vi "SR 8XX read Channel 1&2_Scale.vi"(5 "enable auto?":bool, 6 "read data":enum16{"None", "X Y", "X only"}(ring), 7 "830":bool, 8 "channel":enum16{"R ", "X channel only", "Y channel only"}(ring), 9 "parameters_x":dbl[](array[numeric])=[1.0, 0.95, 0.05, 1e-07, 0.0] format="%.2e", 10 "Point #":i32, 11 "Instrument Address":refnum<visa-resource-name>="GPIB1::4::INSTR") -> (0 "changed range":u8, 1 "changed":bool, 2 "Data":dbl[](array[numeric]) format="%.2e", 3 "CH Output":dbl[](array[numeric]) format="%.2e", 4 "error in (no error) 2":errorcluster)   [LabVIEW 2019]
doc: "This VI reads two channels of the PAR 5210 lockin. It will not work for the 5208. The output is an array of values. The input is the numeric GPIB address.\nScott Hannahs, F. Bitter National Magnet Lab, May 1993"
panel:
  out "original sensitivity":dbl format="%#_2e"
  out "In range":bool
  out "lower limit":dbl format="%#_6e"
  out "upper limit":dbl format="%#_6e"
  out "Y-chanel AO":dbl format="%#_3e"
  out "X-chanel AO":dbl format="%#_3e"
  out "signal > sensitivity":bool
  # "865"
  # "lowest\nsensitivity"
  # "upper\nlimit"
  # "lower\nlimit"
  # "wait after change(sec)"
  # "out of range"
  # "signal < sensitivity"
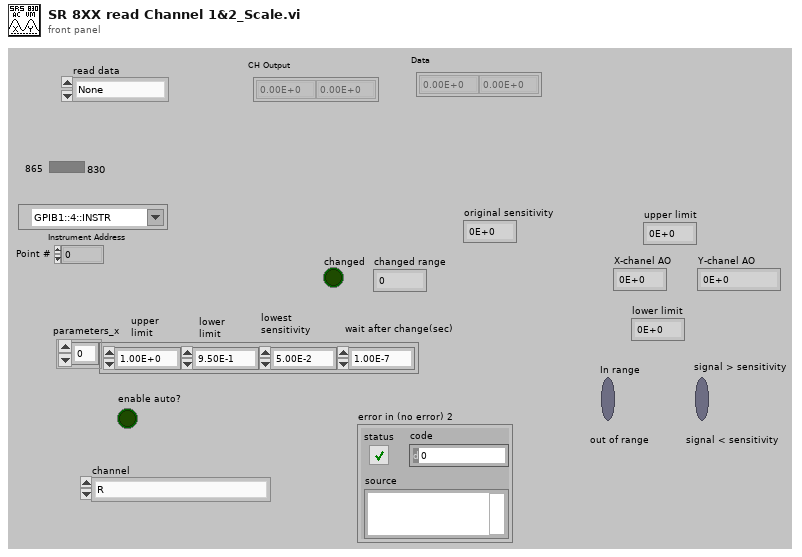
[diagram p1: front panel]
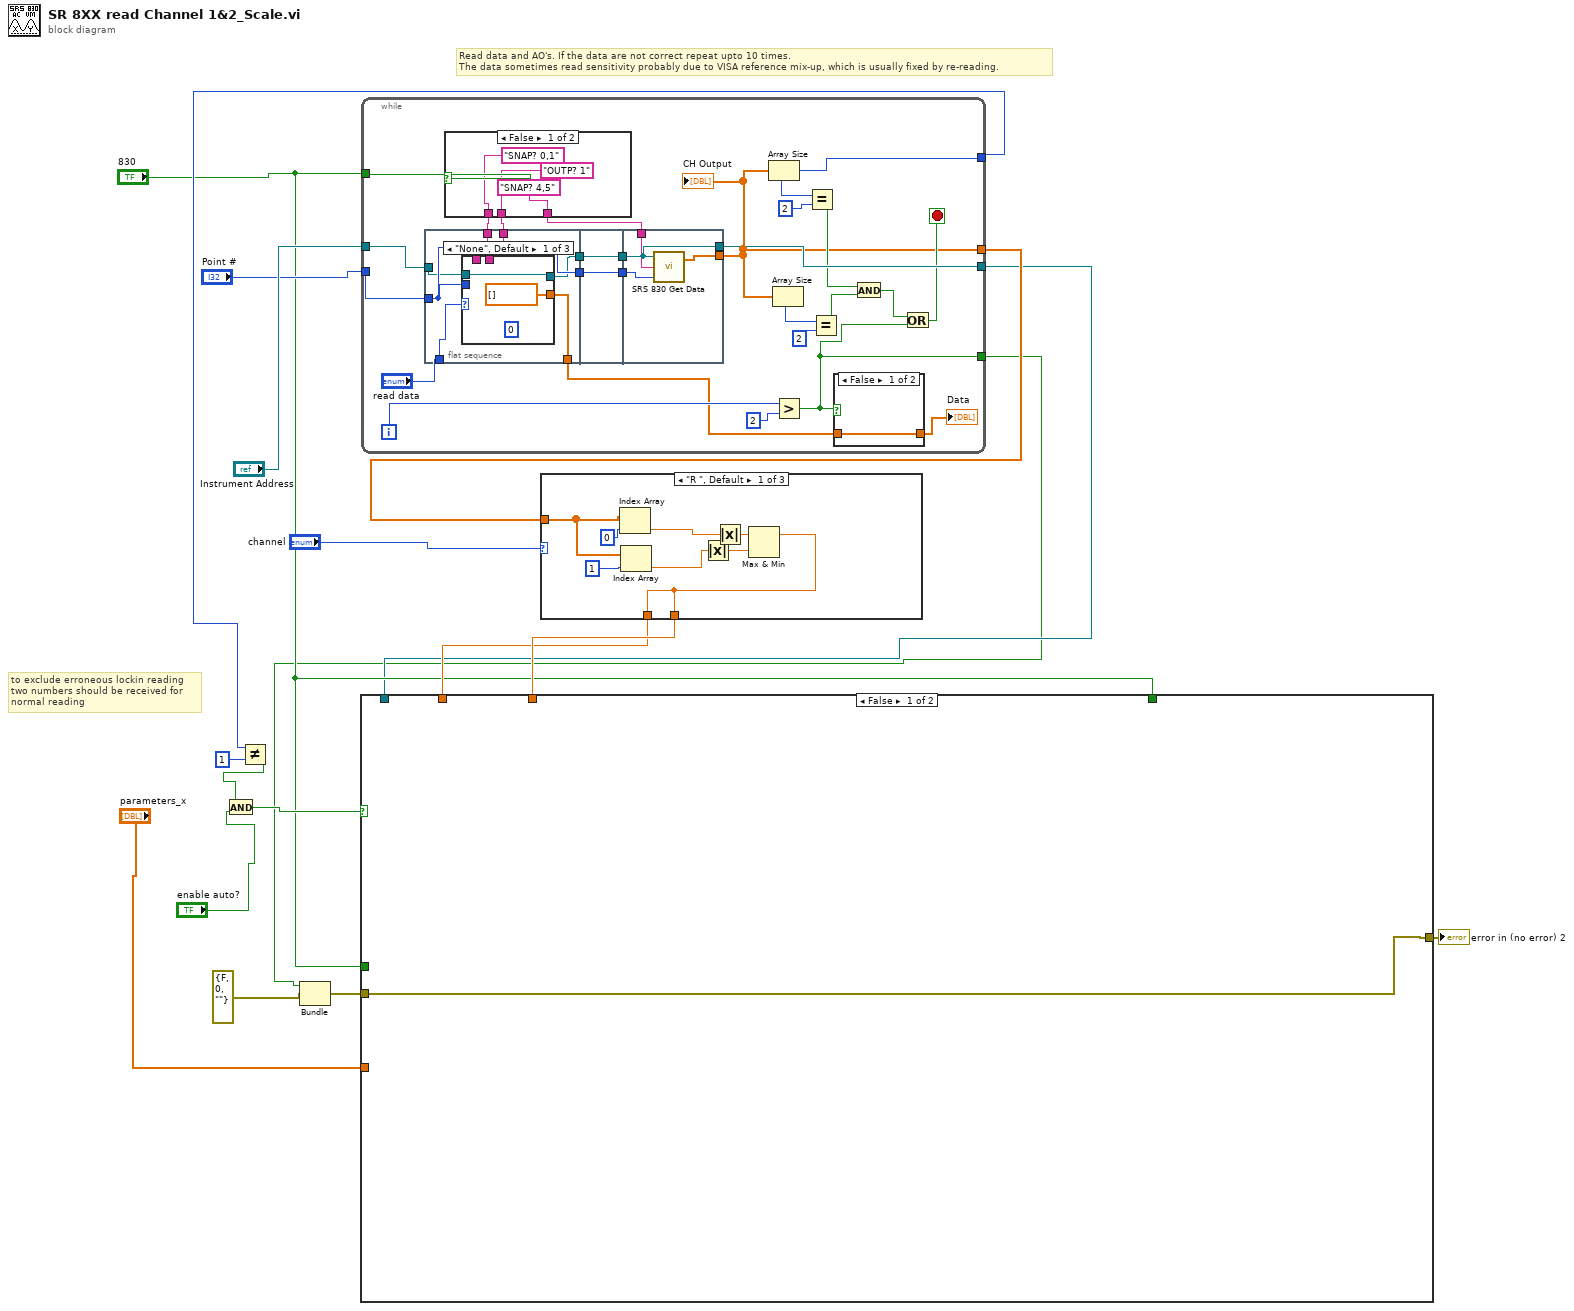
[diagram p0: block diagram]
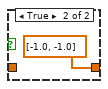
[diagram p2: hidden frame]
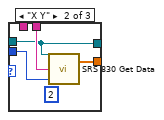
[diagram p3: hidden frame]
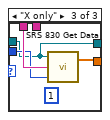
[diagram p4: hidden frame]
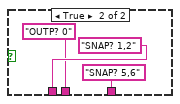
[diagram p5: hidden frame]
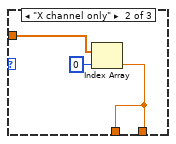
[diagram p6: hidden frame]
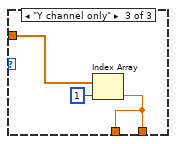
[diagram p7: hidden frame]
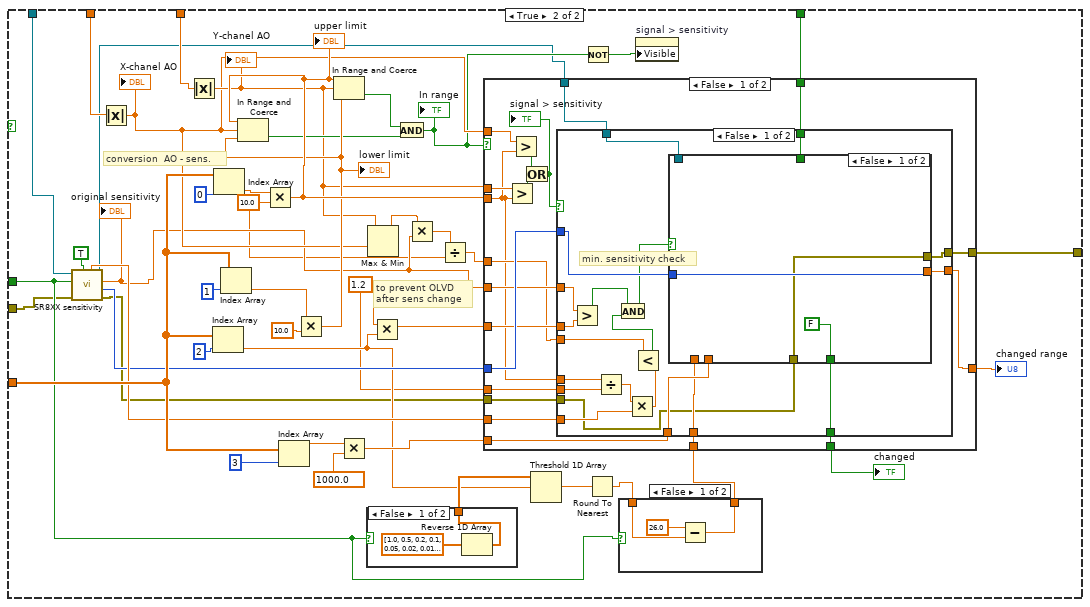
[diagram p8: hidden frame]
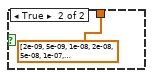
[diagram p10: hidden frame]
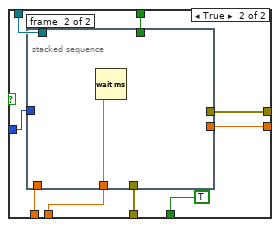
[diagram p11: hidden frame]
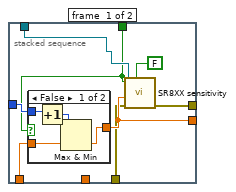
[diagram p12: hidden frame]
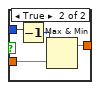
[diagram p13: hidden frame]
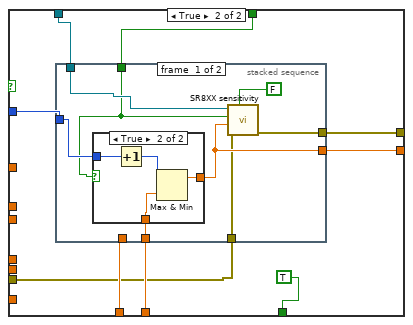
[diagram p14: hidden frame]
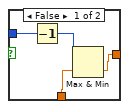
[diagram p15: hidden frame]
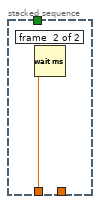
[diagram p16: hidden frame]
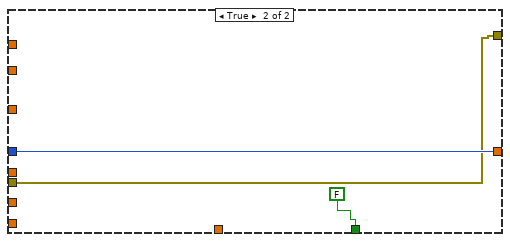
[diagram p17: hidden frame]
diagram:
  # "Read data and AO's. If the data are not correct repeat upto 10 times.\nThe data sometimes read sensitivity probably due to VISA reference mix-up, which is usually fixed by re-reading."
  # "to exclude erroneous lockin reading\ntwo numbers should be received for\nnormal reading"
  n1 = while {
    tunnel: [w22] -> w13
    tunnel: "Instrument Address" -> [w39]
    tunnel: [w43] -> w12
    tunnel: "Point #" -> [w41]
    tunnel: "830" -> [w40]
    tunnel: [w31] -> w5
    tunnel: [w19] -> w1
    i -> [w27]
    stop <- w24 stop-if-true
    n2 = flat-sequence {
      tunnel: w41 -> [w53]
      tunnel: [w53] -> w35
      tunnel: w39 -> [w52]
      tunnel: [w48] -> w33
      tunnel: w38 -> [w51]
      tunnel: "read data" -> [w50]
      tunnel: w36 -> [w49]
      tunnel: [w47] -> w20
      tunnel: w35 -> [w65]
      tunnel: [w65] -> w34
      tunnel: w33 -> [w64]
      tunnel: [w64] -> w32
      tunnel: w44 -> [w69]
      tunnel: [w68] -> w22
      tunnel: w34 -> [w67]
      tunnel: w32 -> [w66]
      tunnel: [w66] -> w31
      frame #0 {
        n3 = case shown="\"None\", Default" w50 {
          tunnel: w53 -> [_ w59 w62]
          tunnel: w52 -> [w55 w57 w61]
          tunnel: w51 -> [_ w58 _]
          tunnel: w49 -> [_ _ w63]
          tunnel: [w55 w57 w61] -> w48
          tunnel: [dbl[] [] ("SRS 830 Output") w56 w60] -> w47
          frame "None", Default {
            (unwired) 0 ("y")
          }
          frame "X Y" {
            (unwired) 2 ("y")
            n4 = call "SRS 830 Get Data.vi"("Point #"=w59, "Command String"=w58, "Instrument Address"=w57) -> ("SRS 830 Output"=w56:dbl[])  [unwired: 1 out]
          }
          frame "X only" {
            (unwired) 1 ("y")
            n5 = call "SRS 830 Get Data.vi"("Point #"=w62, "Command String"=w63, "Instrument Address"=w61) -> ("SRS 830 Output"=w60:dbl[])  [unwired: 1 out]
          }
        }
      }
      frame #1 {
      }
      frame #2 {
        n6 = call "SRS 830 Get Data.vi"("Point #"=w67, "Command String"=w69, "Instrument Address"=w66) -> ("SRS 830 Output"=w68:dbl[])  [unwired: 1 out]
      }
    }
    n7 = case shown="False" w40 {
      tunnel: ["SNAP? 4,5" "SNAP? 5,6"] -> w44
      tunnel: ["SNAP? 0,1" "SNAP? 1,2"] -> w38
      tunnel: ["OUTP? 1" "OUTP? 0"] -> w36
      frame False {
      }
      frame True {
      }
    }
    n8 = Array Size(array=w22) -> (size(s)=w43:i32)
    n9 = Array Size(array=w22) -> (size(s)=w30:i32)
    n10 = Greater?(x=w27, y=2) -> (0:w19:bool)
    n11 = Equal?(x=w43, y=2) -> (x = y?=w29:bool)
    n12 = Equal?(x=w30, y=2) -> (x = y?=w28:bool)
    n13 = case shown="False" w19 {
      tunnel: [w45 dbl[] [-1.0, -1.0] ("SRS 830 Output")] -> w23
      tunnel: w20 -> [w45 _]
      frame False {
      }
      frame True {
      }
    }
    "Data" <- w23
    n14 = And(x=w29, y=w28) -> (x .and. y?=w25:bool)
    n15 = Or(x=w25, y=w19) -> (x .or. y?=w24:bool)
    "CH Output" <- w22
  }
  n16 = Not Equal?(x=w12, y=1) -> (x != y?=w10:bool)
  n17 = And(x=w10, y="enable auto?") -> (x .and. y?=w9:bool)
  n18 = Bundle(cluster=errorcluster {"status"=FALSE, "code"=0, "source"=""} ("error in (no error) 2"), "status"=w1) -> (w3:errorcluster)  [unwired: 2 in]
  n19 = case shown="\"R \", Default" "channel" {
    tunnel: w13 -> [w81 w85 w88]
    tunnel: [w76 w84 w87] -> w16
    tunnel: [w76 w84 w87] -> w15
    frame "R ", Default {
      n20 = Index Array(array=w81, index=0) -> (element=w80:dbl)
      n21 = Index Array(array=w81, index=1) -> (element=w79:dbl)
      n22 = Absolute Value(x=w79) -> (abs(x)=w77:dbl)
      n23 = Absolute Value(x=w80) -> (abs(x)=w78:dbl)
      n24 = Max & Min(x=w78, y=w77) -> (max(x,y)=w76:dbl)  [unwired: 1 out]
    }
    frame "X channel only" {
      n25 = Index Array(array=w85, index=0) -> (element=w84:dbl)
    }
    frame "Y channel only" {
      n26 = Index Array(array=w88, index=1) -> (element=w87:dbl)
    }
  }
  n27 = case shown="False" w9 {
    tunnel: "parameters_x" -> [_ w121]
    tunnel: w5 -> [_ w126]
    tunnel: w16 -> [_ w115]
    tunnel: w15 -> [_ w114]
    tunnel: "830" -> [_ w95]
    tunnel: "830" -> [_ w98]
    tunnel: [w90 w92] -> w4
    tunnel: w3 -> [w90 w91]
    frame False {
    }
    frame True {
      w100 = 10.0 ("y")
      w99 = 1.2 ("x")
      # "conversion  AO - sens."
      # "to prevent OLVD\nafter sens change"
      n28 = call "SR8XX sensitivity.vi"("Instrument Address"=w126, "830"=w95, "error in (no error)"=w91, "read"=TRUE) -> ("one step lower sensitivity"=w120:dbl, "dup VISA session"=w94:refnum<visa-resource-name>, "sensitivity"=w103:dbl, "range number"=w113:i32, "error in (no error) 2"=w93:errorcluster)  [unwired: 1 in, 1 out]
      "original sensitivity" <- w103
      n29 = Absolute Value(x=w114) -> (abs(x)=w118:dbl)
      "X-chanel AO" <- w118
      n30 = Absolute Value(x=w115) -> (abs(x)=w119:dbl)
      "Y-chanel AO" <- w119
      n31 = Index Array(array=w121, index=2 ("Index")) -> (element=w108:dbl)
      n32 = Index Array(array=w121, index=0 ("Index")) -> (element=w112:dbl)
      n33 = Index Array(array=w121, index=1 ("Index")) -> (element=w133:dbl)
      n34 = Multiply(x=w112, y=w100) -> (x*y=w124:dbl)
      "upper limit" <- w124
      n35 = Index Array(array=w121, index=3 ("Index")) -> (element=w131:dbl)
      n36 = Multiply(x=w133, y=10.0) -> (x*y=w123:dbl)
      "lower limit" <- w123
      n37 = In Range and Coerce(upper limit=w124, x=w118, lower limit=w123) -> (In Range?=w122:bool)  [unwired: 1 out]
      n38 = In Range and Coerce(upper limit=w124, x=w119, lower limit=w123) -> (In Range?=w127:bool)  [unwired: 1 out]
      n39 = Multiply(x=w131, y=sgl 1000.0) -> (x*y=w129:dbl)
      n40 = case shown="False" w95 {
        tunnel: [w140 dbl[] [2e-09, 5e-09, 1e-08, 2e-08, 5e-08, 1e-07, 2.0000000000000002e-07, 5.000000000000001e-07, 1.0000000000000002e-06, 2.0000000000000003e-06, 5.000000000000001e-06, 1.0000000000000003e-05, 2e-05, 5e-05, 0.0001, 0.0002, 0.0005, 0.001, 0.002, 0.005, 0.01, 0.02, 0.05, 0.1, 0.2, 0.5, 1.0] ("Array")] -> w110
        frame False {
          n41 = Reverse 1D Array(array=dbl[] [1.0, 0.5, 0.2, 0.1, 0.05, 0.02, 0.01, 0.005, 0.002, 0.001, 0.0005, 0.0002, 0.0001, 5e-05, 2e-05, 1.0000000000000003e-05, 5.000000000000001e-06, 2.0000000000000003e-06, 1.0000000000000002e-06, 5.000000000000001e-07, 2.0000000000000002e-07, 1e-07, 5e-08, 2e-08, 1e-08, 5e-09, 2e-09] ("reversed array")) -> (reversed array=w140:dbl[])
        }
        frame True {
        }
      }
      n42 = Max & Min(x=w119, y=w118) -> (max(x,y)=w104:dbl)  [unwired: 1 out]
      n43 = Multiply(x=w99, y=w108) -> (x*y=w111:dbl)
      n44 = And(x=w127, y=w122) -> (x .and. y?=w106:bool)
      "In range" <- w106
      n45 = Multiply(x=w104, y=w103) -> (x*y=w102:dbl)
      n46 = Divide(x=w102, y=w100) -> (x/y=w101:dbl)
      n47 = Threshold 1D Array(2:w108, 3:w110) -> (0:w109:dbl)  [unwired: 1 in]
      n48 = Not(x=w106) -> (.not. x?=w107:bool)
      n49 = Round To Nearest(number=w109) -> (nearest integer value=w97:dbl)
      n50 = case shown="False" w95 {
        tunnel: [w136 w139] -> w96
        tunnel: w97 -> [w138 w139]
        frame False {
          n51 = Subtract(x=26.0, y=w138) -> (x-y=w136:dbl)
        }
        frame True {
        }
      }
      n52 = case shown="False" w106 {
        tunnel: w124 -> [w147 _]
        tunnel: w94 -> [w162 _]
        tunnel: w113 -> [w161 w240]
        tunnel: w119 -> [w152 _]
        tunnel: w129 -> [w160 _]
        tunnel: w103 -> [w159 _]
        tunnel: w111 -> [w158 _]
        tunnel: w118 -> [w155 _]
        tunnel: w120 -> [w153 _]
        tunnel: w101 -> [w151 _]
        tunnel: [w150 w240] -> w117
        tunnel: [w149 FALSE] -> w116
        tunnel: w96 -> [w148 _]
        tunnel: w99 -> [w146 _]
        tunnel: w98 -> [w145 _]
        tunnel: w93 -> [w144 w238]
        tunnel: [w143 w238] -> w92
        frame False {
          n53 = Greater?(x=w152, y=w147) -> (0:w157:bool)
          n54 = Greater?(x=w155, y=w147) -> (0:w154:bool)
          n55 = Or(x=w154, y=w157) -> (x .or. y?=w156:bool)
          "signal > sensitivity" <- w156
          n56 = case shown="False" w156 {
            tunnel: w162 -> [w182 w220]
            tunnel: w161 -> [w181 w219]
            tunnel: w160 -> [w180 w218]
            tunnel: w159 -> [w179 _]
            tunnel: w158 -> [w178 _]
            tunnel: w153 -> [w175 _]
            tunnel: w151 -> [w173 _]
            tunnel: [w171 w217] -> w150
            tunnel: [w170 TRUE] -> w149
            tunnel: w148 -> [w168 w215]
            tunnel: w147 -> [w167 _]
            tunnel: w146 -> [w166 _]
            tunnel: w145 -> [w165 w214]
            tunnel: w144 -> [w164 w213]
            tunnel: [w163 w212] -> w143
            frame False {
              # "min. sensitivity check"
              n57 = Greater?(x=w179, y=w178) -> (0:w177:bool)
              n58 = Divide(x=w167, y=w166) -> (x/y=w169:dbl)
              n59 = Multiply(x=w169, y=w175) -> (x*y=w174:dbl)
              n60 = Less?(x=w173, y=w174) -> (x < y?=w172:bool)
              n61 = And(x=w177, y=w172) -> (x .and. y?=w176:bool)
              n62 = case shown="False" w176 {
                tunnel: w182 -> [_ w194]
                tunnel: w181 -> [w185 w193]
                tunnel: w180 -> [_ w192]
                tunnel: [w185 w191] -> w171
                tunnel: [FALSE TRUE] -> w170
                tunnel: w168 -> [_ w189]
                tunnel: w165 -> [_ w188]
                tunnel: w164 -> [w183 w187]
                tunnel: [w183 w186] -> w163
                frame False {
                }
                frame True {
                  n63 = stacked-sequence {
                    tunnel: w194 -> [w200 _]
                    tunnel: w193 -> [w202 _]
                    tunnel: w192 -> [_ w211]
                    tunnel: [w199 _] -> w191
                    tunnel: w189 -> [w198 _]
                    tunnel: w188 -> [w197 _]
                    tunnel: w187 -> [w196 _]
                    tunnel: [w195 _] -> w186
                    frame #0 {
                      n64 = case shown="False" w197 {
                        tunnel: w202 -> [w206 w210]
                        tunnel: [w203 w208] -> w199
                        tunnel: w198 -> [w204 w207]
                        frame False {
                          n65 = Increment(x=w206) -> (x+1=w205:i32)
                          n66 = Max & Min(x=w205, y=w204) -> (min(x,y)=w203:dbl)  [unwired: 1 out]
                        }
                        frame True {
                          n67 = Decrement(x=w210) -> (x-1=w209:i32)
                          n68 = Max & Min(x=w209, y=w207) -> (max(x,y)=w208:dbl)  [unwired: 1 out]
                        }
                      }
                      n69 = call "SR8XX sensitivity.vi"("Instrument Address"=w200, "830"=w197, "set range index"=w199, "error in (no error)"=w196, "read"=FALSE ("set")) -> ("error in (no error) 2"=w195:errorcluster)  [unwired: 5 out]
                    }
                    frame #1 {
                      n70 = Wait (ms)(milliseconds to wait=w211) -> ()  [unwired: 1 out]
                    }
                  }
                }
              }
            }
            frame True {
              n71 = stacked-sequence {
                tunnel: w220 -> [w227 _]
                tunnel: w219 -> [w228 _]
                tunnel: w218 -> [_ w237]
                tunnel: [w224 _] -> w217
                tunnel: w215 -> [w225 _]
                tunnel: w214 -> [w223 _]
                tunnel: w213 -> [w222 _]
                tunnel: [w221 _] -> w212
                frame #0 {
                  n72 = case shown="True" w223 {
                    tunnel: w228 -> [w232 w236]
                    tunnel: w225 -> [w230 w234]
                    tunnel: [w229 w233] -> w224
                    frame False {
                      n73 = Decrement(x=w232) -> (x-1=w231:i32)
                      n74 = Max & Min(x=w231, y=w230) -> (min(x,y)=w229:dbl)  [unwired: 1 out]
                    }
                    frame True {
                      n75 = Increment(x=w236) -> (x+1=w235:i32)
                      n76 = Max & Min(x=w235, y=w234) -> (max(x,y)=w233:dbl)  [unwired: 1 out]
                    }
                  }
                  n77 = call "SR8XX sensitivity.vi"("Instrument Address"=w227, "830"=w223, "set range index"=w224, "error in (no error)"=w222, "read"=FALSE ("set")) -> ("error in (no error) 2"=w221:errorcluster)  [unwired: 5 out]
                }
                frame #1 {
                  n78 = Wait (ms)(milliseconds to wait=w237) -> ()  [unwired: 1 out]
                }
              }
            }
          }
        }
        frame True {
        }
      }
      "changed range" <- w117
      "changed" <- w116
      n79 = property on="signal > sensitivity" class="Bool (strict)"("Visible"=w107) -> ()  [unwired: 2 in, 2 out]
    }
  }
  "error in (no error) 2" <- w4
